vi "Create Stimulus Session.vi"(8 "Error In":errorcluster, 9 "Session Name (CSVPlayerSession)":string="CSVPlayerSession", 10 "Parameter Defaults":string[][](array[string]), 11 "Seq":path) -> (0 "Error Out":errorcluster, 1 "Seq Name":string, 3 "Stim Session Ref":T1)   [LabVIEW 2011]
uses:
  <vilib>/NI Veristand/Execution/SequenceExecutionInterface/Stimulus Profile Session Ref.ctl
  NationalInstruments.VeriStand.ClientAPI
  <vilib>/NI Veristand/Execution/SequenceExecutionInterface/Create Sequence Parameter Assignment (Channel).vi
  <vilib>/NI Veristand/Execution/SequenceExecutionInterface/NI_VS Sequence Execution Interface.lvlib
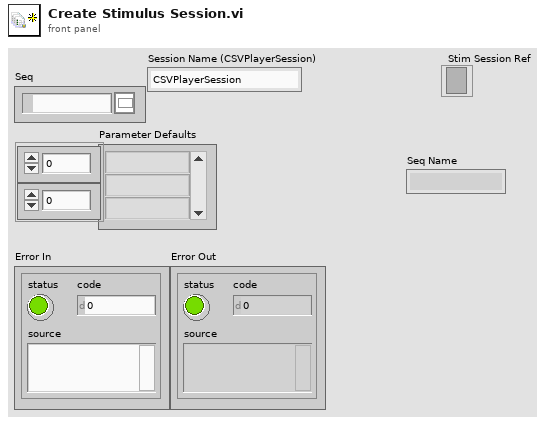
[diagram p1: front panel]
types:
  T1 = typedef "NI_VS Sequence Execution Interface.lvlib/Stimulus Profile Session Ref.ctl" = refnum<k24>
  T2 = typedef "NI_VS Sequence Execution Interface.lvlib/Sequence Input Assignment Ref.ctl" = refnum<k24>
  T3 = typedef "NI_VS Sequence Execution Interface.lvlib/Sequence Call Ref.ctl" = refnum<k24>
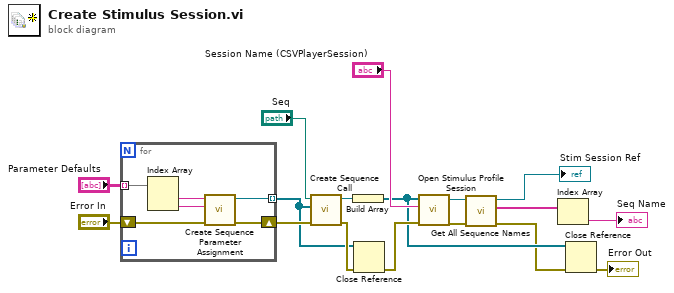
[diagram p0: block diagram]
diagram:
  n1 = for {
    tunnel: "Parameter Defaults" -> [w23] mode=indexing
    shift-right: [w19] -> w14
    shift-left: "Error In" -> [w20]
    tunnel: [w18] -> w9 mode=indexing
    n2 = Index Array(array=w23) -> (element #1=w22:string, element #2=w21:string)  [unwired: 2 in]
    n3 = call-poly <vilib>:"Create Sequence Parameter Assignment.vi"("error in (no error)"=w20, "Channel"=w21, "Parameter Name"=w22) -> ("error out"=w19:errorcluster, "Sequence Parameter Assignment Ref"=w18:T2)  [unwired: 7 in]
  }
  n4 = call <vilib>:"Create Sequence Call.vi"("error in (no error)"=w14, "Parameter Assignments"=w9, "Sequence File Path"="Seq") -> ("error out"=w11:errorcluster, "Sequence Call Ref"=w13:T3)  [unwired: 7 in]
  n5 = Build Array(w13) -> (w7:T3[])
  n6 = Close Reference(reference=w9, error in (no error)=w11) -> (error out=w10:errorcluster)
  n7 = call <vilib>:"Open Stimulus Profile Session.vi"("error in (no error)"=w10, "Session Name"="Session Name (CSVPlayerSession)", "Sequence Calls"=w7) -> ("error out"=w6:errorcluster, "Session Ref"=w5:T1)  [unwired: 7 in]
  n8 = call <vilib>:"Get All Sequence Names.vi"("error in (no error)"=w6, "Session Ref in"=w5) -> ("error out"=w3:errorcluster, "Sequence Names out"=w2:string[], "Session Ref out"=→"Stim Session Ref":T1)  [unwired: 7 in]
  n9 = Index Array(array=w2) -> (element=→"Seq Name":string)  [unwired: 1 in]
  n10 = Close Reference(reference=w7, error in (no error)=w3) -> (error out=→"Error Out":errorcluster)
